vi "Read_sig_file.vi"() -> ()   [LabVIEW 2015]
panel:
  out "size (in bytes)":i64
  out "Waveform Graph":i16[][](graph)
  in  "start path":path=path "C:/Program Files (x86)/Gage/CompuScope/CompuScope LabVIEW SDK/Main/Signals"
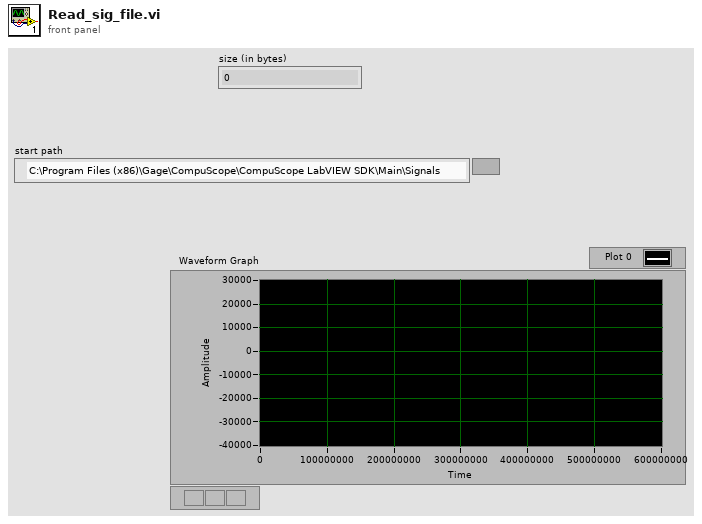
[diagram p1: front panel]
types:
  T1 = enum16{"big-endian, network order", "native, host order", "little-endian"}
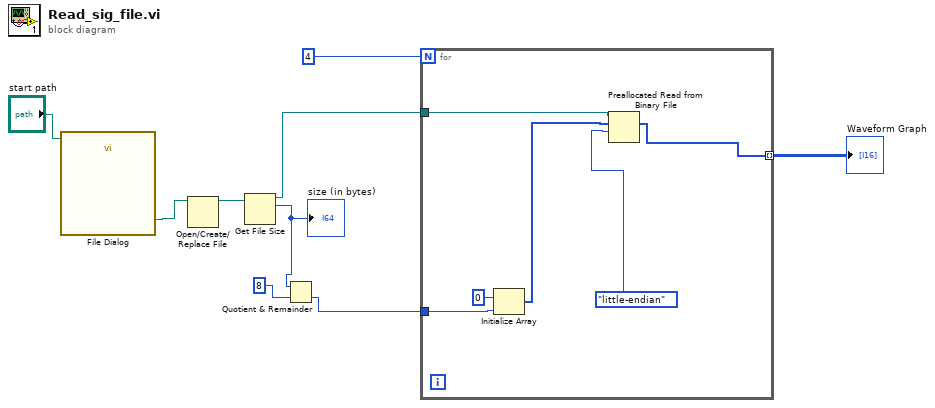
[diagram p0: block diagram]
diagram:
  n1 = call "File Dialog"("start path"="start path") -> ("selected path"=w8:path)  [unwired: 11 in, 3 out]
  n2 = Open/Create/Replace File(file path (use dialog)=w8) -> (refnum out=w7:refnum<file>)  [unwired: 5 in, 2 out]
  n3 = Get File Size(file=w7) -> (refnum out=w6:refnum<file>, size (in bytes)=w5:i64)  [unwired: 1 in, 1 out]
  "size (in bytes)" <- w5
  n4 = Quotient & Remainder(x=w5, y=i64 8) -> (floor(x/y)=w4:i64)  [unwired: 1 out]
  n5 = for {
    N: i64 4 ("y") -> [_]
    tunnel: w6 -> [w15]
    tunnel: w4 -> [w14]
    tunnel: [w10] -> w3 mode=indexing
    n6 = Initialize Array(i16 0 ("element"), w14) -> (w12:i16[])
    n7 = Preallocated Read from Binary File(5:T1."little-endian" ("byte order (0:big-endian, network order)"), 6:w12, 7:w15) -> (2:w10:i16[])  [unwired: 1 in, 3 out]
  }
  "Waveform Graph" <- w3
